vi "FPS_Calculator.vi"() -> (3 "FPS":dbl)   [LabVIEW 2016]
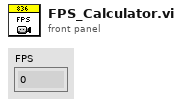
[diagram p1: front panel]
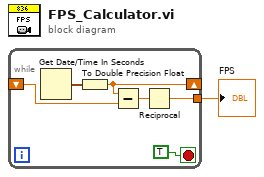
[diagram p0: block diagram]
diagram:
  n1 = while {
    shift-right: [w2] -> _
    shift-left: _ -> [w6]
    tunnel: [w3] -> w1
    stop <- TRUE stop-if-true
    n2 = Get Date/Time In Seconds() -> (seconds since 1Jan1904=w7:timestamp)
    n3 = To Double Precision Float(number=w7) -> (double precision float=w2:dbl)
    n4 = Subtract(x=w2, y=w6) -> (x-y=w4:dbl)
    n5 = Reciprocal(x=w4) -> (1/x=w3:dbl)
  }
  "FPS" <- w1
